vi "ReleaseControl.vi"(8 "error in (no error)":errorcluster, 10 "locked by":string, 11 "BME_DG_System in":refnum<class "BME_DG_System.lvclass">) -> (0 "error out":errorcluster, 1 "level out":T1, 2 "locked by out":string, 3 "BME_DG_System out":refnum<class "BME_DG_System.lvclass">, 5 "Success?":bool)   [LabVIEW 2009, in "POLARIS BME DG.lvlib" / "BME_DG_System.lvclass"]
uses:
  BME_DG_System.lvclass
  ControlLevel.ctl
  BME_DG_System.lvclass/BME_DG_System.ctl
  POLARIS BME DG.lvlib
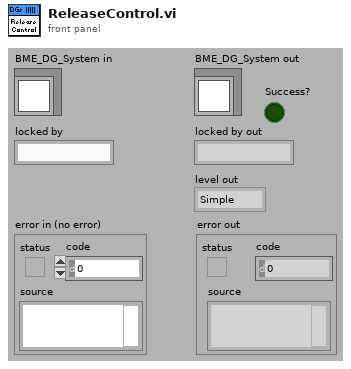
[diagram p1: front panel]
types:
  T1 = typedef "POLARIS BME DG.lvlib/BME_DG_System.lvclass/ControlLevel.ctl" = enum16{"Simple", "Expert", "Unknown"}
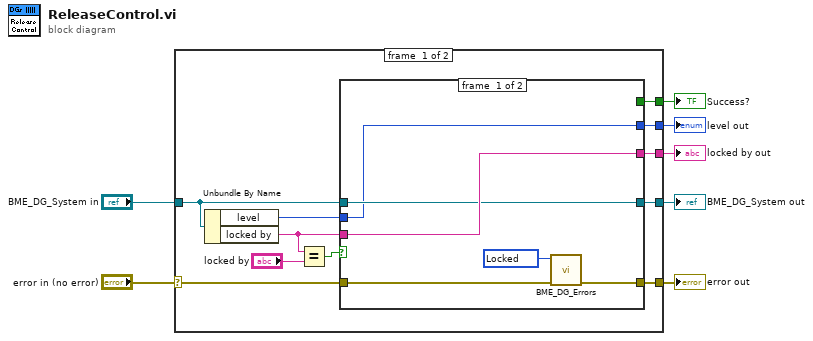
[diagram p0: block diagram]
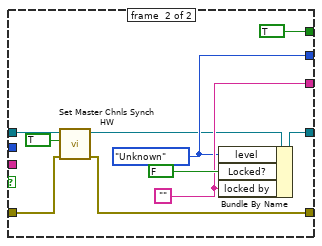
[diagram p2: hidden frame]
diagram:
  n1 = case shown="No Error" "error in (no error)" {
    selector: "error in (no error)" -> [w18 w36]
    tunnel: [w17 w36] -> w6
    tunnel: [w16 w35] -> w4
    tunnel: "BME_DG_System in" -> [w15 w35]
    tunnel: [w14 _] -> w3
    tunnel: [w13 _] -> w2
    tunnel: [w12 _] -> w1
    frame #0 {
      n2 = Unbundle By Name(w15) -> ("level"=w11:T1, "locked by"=w8:string)
      n3 = Equal?(x=w8, y="locked by") -> (x = y?=w10:bool)
      n4 = case shown="True" w10 {
        tunnel: w8 -> [w21 _]
        tunnel: w18 -> [w24 w26]
        tunnel: [w23 w25] -> w17
        tunnel: [w20 w34] -> w16
        tunnel: w15 -> [w20 w29]
        tunnel: [w21 w31] -> w14
        tunnel: [_ TRUE] -> w13
        tunnel: [w19 w30] -> w12
        tunnel: w11 -> [w19 _]
        frame #0 {
          w22 = 503013 items=["Channel refers itself"=503001, "Deadloop"=503002, "Negative Delay"=503003, "Delay Card not found"=503004, "Channel not found"=503005, "Parse Error"=503006, "Not Supported"=503007, "Systen not found"=503008, "To much masters"=503009, "None master in Syterm"=503010, "InterruptError"=503011, "ChnlPeriodeWarning"=503012, "Locked"=503013] ("error")
          n5 = call "BME_DG_Errors.vi"("error in (no error)"=w24, "error"=w22) -> ("error out"=w23:errorcluster)  [unwired: 9 in]
        }
        frame #1 {
          w30 = ControlLevel."Unknown" ("level")
          w31 = ""
          n6 = call-dynamic "Set Master Chnls Synch HW.vi"("error in (no error)"=w26, "Synch?"=TRUE, "BME_DG_System in"=w29) -> ("error out"=w25:errorcluster, "BME_DG_System out"=w28:refnum<class "BME_DG_System.lvclass">)  [unwired: 7 in]
          n7 = Bundle By Name(cluster=w28, "level"=w30, "Locked?"=FALSE, "locked by"=w31) -> (w34:refnum<class "BME_DG_System.lvclass">)
        }
      }
    }
    frame #1 {
    }
  }
  "error out" <- w6
  "BME_DG_System out" <- w4
  "locked by out" <- w3
  "Success?" <- w2
  "level out" <- w1
